vi "Open.vi"(8 "error in (no error)":errorcluster, 10 "Interface_type":T1="DALI", 11 "_Driver_interaction in":refnum<class "_Driver_interaction.lvclass">) -> (0 "error out":errorcluster, 3 "_Driver_interaction out":refnum<class "_Driver_interaction.lvclass">)   [LabVIEW 2014, in "Driver_interaction.lvlib" / "_Driver_interaction.lvclass"]
uses:
  _Driver_interaction.lvclass
  Controls/Interface_type.ctl
  _Driver_interaction.lvclass/_Driver_interaction.ctl
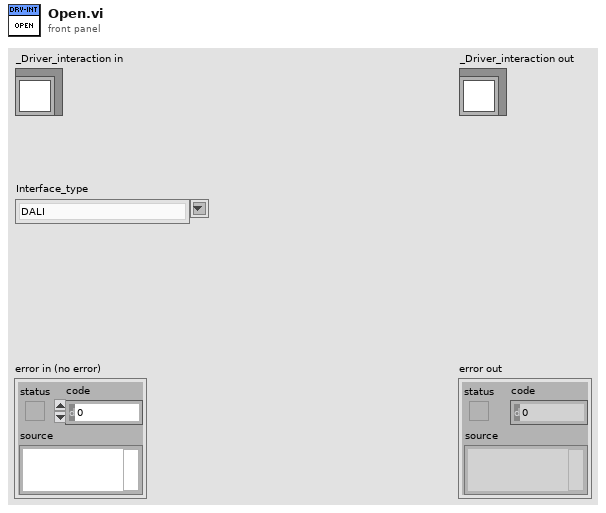
[diagram p1: front panel]
types:
  T1 = typedef "Driver_interaction.lvlib/_Driver_interaction.lvclass/Interface_type.ctl" = string
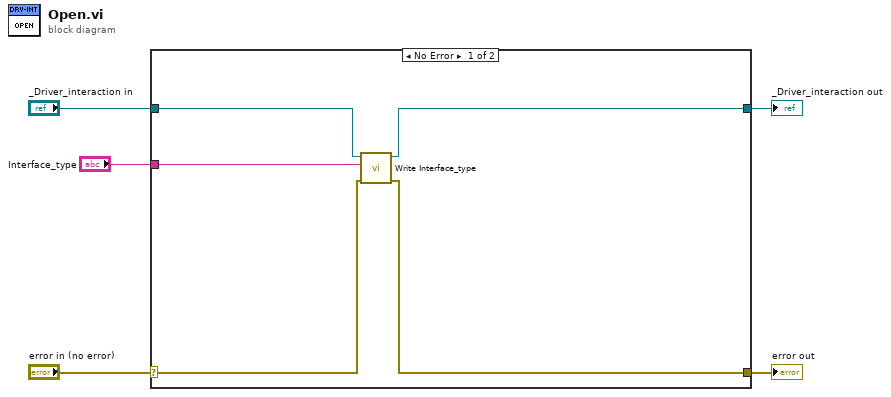
[diagram p0: block diagram]
diagram:
  n1 = case shown="No Error" "error in (no error)" {
    selector: "error in (no error)" -> [w7 w12]
    tunnel: [w6 w12] -> w4
    tunnel: [w8 w11] -> w2
    tunnel: "_Driver_interaction in" -> [w10 w11]
    tunnel: "Interface_type" -> [w9 _]
    frame No Error {
      n2 = call "Write Interface_type.vi"("error in (no error)"=w7, "Interface_type"=w9, "_Driver_interaction in"=w10) -> ("error out"=w6:errorcluster, "_Driver_interaction out"=w8:refnum<class "_Driver_interaction.lvclass">)  [unwired: 7 in]
    }
    frame Error {
    }
  }
  "error out" <- w4
  "_Driver_interaction out" <- w2
